vi "Manage Collision.vi"(11 "Ball-Missile in":refnum<class "Ball-Missile.lvclass">) -> (1 "Remove GB Components out":refnum<class "Game Board Component.lvclass">[](array[class]), 2 "GB Components out":refnum<class "Game Board Component.lvclass">[](array[class]))   [LabVIEW 2021, in "Ball-Missile.lvclass"]
doc: "MIT Licence\nCopyright (c) 2024 David Grollier"
uses:
  Ball-Missile.lvclass
  C:/Users/David/Documents/GameSoccerSpace/Source/Collision/Collision.lvclass
  Game Componants/Game Board Component/Game Board Component.lvclass
  Game Componants/Game Board Component/Movable/Movable.lvclass
  C:/Users/David/Documents/GameSoccerSpace/Source/Game Componants/Game Board Component/Game Board Component.lvclass
  C:/Users/David/Documents/GameSoccerSpace/Source/Game Componants/Game Componants.lvclass
  Game Componants/Game Board Component/Movable/Missile/Missile.lvclass
  Collision.lvclass/Collision.ctl
  Game Componants/Game Board Component/Movable/Movable.lvclass/Movable.ctl
  Game Componants/Game Componants.lvclass/Game Componants.ctl
  Game Componants/Game Componants.lvclass
  Collision.lvclass
  Game Componants/Game Board/Game Board.lvclass
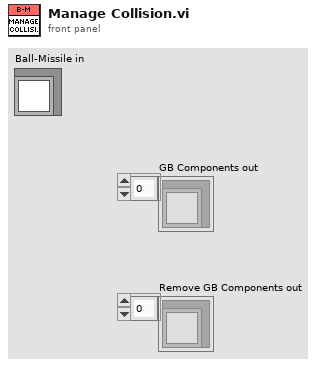
[diagram p1: front panel]
types:
  T1 = typedef "Velocity.ctl" = cluster{"Vx":dbl, "Vy":dbl}
  T2 = typedef "Coordinates.ctl" = cluster{"x":dbl, "y":dbl}
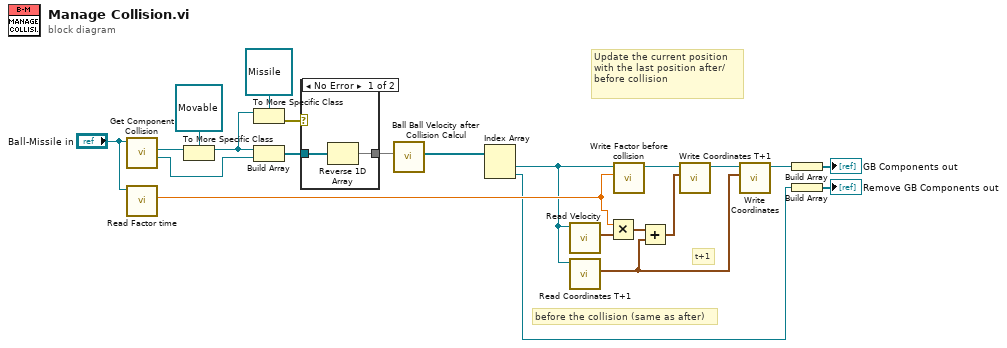
[diagram p0: block diagram]
diagram:
  # "t+1"
  # "before the collision (same as after)"
  # "Update the current position with the last position after/before collision"
  n1 = call "Get Component Collision.vi"("Collision in"="Ball-Missile in") -> ("Movable out"=w21:refnum<class "Movable.lvclass">, "GB Component out"=w20:refnum<class "Game Board Component.lvclass">)  [unwired: 9 in]
  n2 = call "Read Factor time.vi"("Collision in"="Ball-Missile in") -> ("Factor time"=w22:dbl)  [unwired: 10 in]
  n3 = To More Specific Class(target class=refnum<class "Movable.lvclass"> refnum ("specific class reference"), reference=w20) -> (specific class reference=w5:refnum<class "Movable.lvclass">)  [unwired: 1 in, 1 out]
  n4 = To More Specific Class(target class=refnum<class "Missile.lvclass"> refnum ("Missile.lvclass"), reference=w5) -> (error out=w3:errorcluster)  [unwired: 1 in, 1 out]
  n5 = Build Array(w5, w21) -> (w2:refnum<class "Movable.lvclass">[])
  n6 = case shown="No Error" w3 {
    tunnel: w2 -> [w24 w25]
    tunnel: [w23 w25] -> w1
    frame No Error {
      n7 = Reverse 1D Array(array=w24) -> (reversed array=w23:refnum<class "Movable.lvclass">[])
    }
    frame Error {
    }
  }
  n8 = call "Ball Ball Velocity after Collision Calcul.vi"("Movables in"=w1) -> ("Movables out"=w18:refnum<class "Movable.lvclass">[])  [unwired: 10 in]
  n9 = Index Array(array=w18) -> (element #1=w17:refnum<class "Movable.lvclass">, element #2=w10:refnum<class "Movable.lvclass">)  [unwired: 2 in]
  n10 = call-dynamic "Read Velocity.vi"("Movable in"=w17) -> ("Velocity"=w15:T1)  [unwired: 10 in]
  n11 = call "Read Coordinates T+1.vi"("Movable in"=w17) -> ("Coordinates"=w14:T2)  [unwired: 10 in]
  n12 = Multiply(x=w22, y=w15) -> (x*y=w16:T1)
  n13 = call "Write Factor before collision.vi"("Factor before collision"=w22, "Movable in"=w17) -> ("Movable out"=w12:refnum<class "Movable.lvclass">)  [unwired: 9 in]
  n14 = Add(x=w16, y=w14) -> (x+y=w13:T1)
  n15 = call "Write Coordinates T+1.vi"("Coordinates"=w13, "Movable in"=w12) -> ("Movable out"=w11:refnum<class "Movable.lvclass">)  [unwired: 9 in]
  n16 = call "Write Coordinates.vi"("Coordinates"=w14, "Game Componants in"=w11) -> ("Game Componants out"=w9:refnum<class "Movable.lvclass">)  [unwired: 9 in]
  n17 = Build Array(w9) -> (→"GB Components out":refnum<class "Movable.lvclass">[])
  n18 = Build Array(w10) -> (→"Remove GB Components out":refnum<class "Movable.lvclass">[])
